vi "Configure Hardware.vi"(8 "error in (no error)":errorcluster, 11 "Cluster":T1={"Camera.lvclass"=refnum, "InClusTiming 2"={"Pixelclock"=24, "Exposure"=46.39115, "ExposureTimeBase"=2, "Framerate"=14.99615, "TriggerMode"=0}, "ROI"={"PosX"=0, "PosY"=0, "Width"=0, "Height"=0}, "File Path Control"=path "", "mirror.lvclass"=refnum} {"InClusTiming 2"."TriggerMode" items=["Auto", "Software", "External sequence start ", "External exposure control"]; "InClusTiming 2"."ExposureTimeBase" items=["nanoseconds", "microseconds", "milliseconds"]; "InClusTiming 2"."Pixelclock" min=1 max=400 step=1 scale=0.05915..400.0 scale format="%#.3g"; "InClusTiming 2"."Framerate" min=0.05915 max=2000.0 step=1.0 scale=0.05915..100.0 scale format="%#.3g"; "InClusTiming 2"."Exposure" min=0.05915 max=2000.0 step=1.0 scale=0.05915..100.0 scale format="%#.3g"}) -> (0 "error out":errorcluster, 2 "initialized array":sgl[][](array[numeric]) format="%.2f", 3 "Cluster 2":T1={"Camera.lvclass"=refnum, "InClusTiming 2"={"Pixelclock"=24, "Exposure"=46.39115, "ExposureTimeBase"=2, "Framerate"=14.99615, "TriggerMode"=0}, "ROI"={"PosX"=0, "PosY"=0, "Width"=0, "Height"=0}, "File Path Control"=path "", "mirror.lvclass"=refnum} {"InClusTiming 2"."TriggerMode" items=["Auto", "Software", "External sequence start ", "External exposure control"]; "InClusTiming 2"."ExposureTimeBase" items=["nanoseconds", "microseconds", "milliseconds"]; "InClusTiming 2"."Pixelclock" min=1 max=400 step=1 scale=0.05915..400.0 scale format="%#.3g"; "InClusTiming 2"."Framerate" min=0.05915 max=2000.0 step=1.0 scale=0.05915..100.0 scale format="%#.3g"; "InClusTiming 2"."Exposure" min=0.05915 max=2000.0 step=1.0 scale=0.05915..100.0 scale format="%#.3g"})   [LabVIEW 2020, in "Acquisition.lvlib"]
doc: "Configure the hardware."
uses:
  Acquisition.lvlib
  HardwareConfiguration.ctl
  CLASS/Image Acquisition Class/Camera.lvclass
  MIRROR/mirror.lvclass
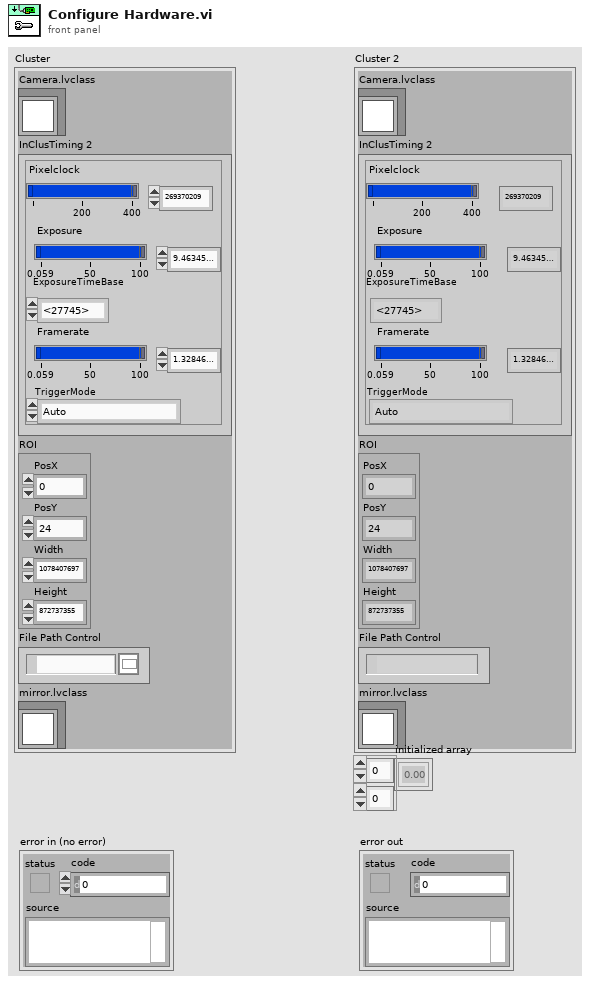
[diagram p1: front panel]
types:
  T1 = typedef "Acquisition.lvlib/HardwareConfiguration.ctl" = cluster{"Camera.lvclass":refnum<class "Camera.lvclass">, "InClusTiming 2":cluster{"Pixelclock":i32, "Exposure":dbl, "ExposureTimeBase":u16, "Framerate":dbl, "TriggerMode":u16}, "ROI":cluster{"PosX":i32, "PosY":i32, "Width":i32, "Height":i32}, "File Path Control":path, "mirror.lvclass":refnum<class "mirror.lvclass">}
  T2 = enum16{"Initialisation", "Calcul CdG a", "Calcul CdG b"}
  T3 = cluster{"Pixelclock":i32, "Exposure":dbl, "ExposureTimeBase":u16, "Framerate":dbl, "TriggerMode":u16}
  T4 = cluster{"PosX":i32, "PosY":i32, "Width":i32, "Height":i32}
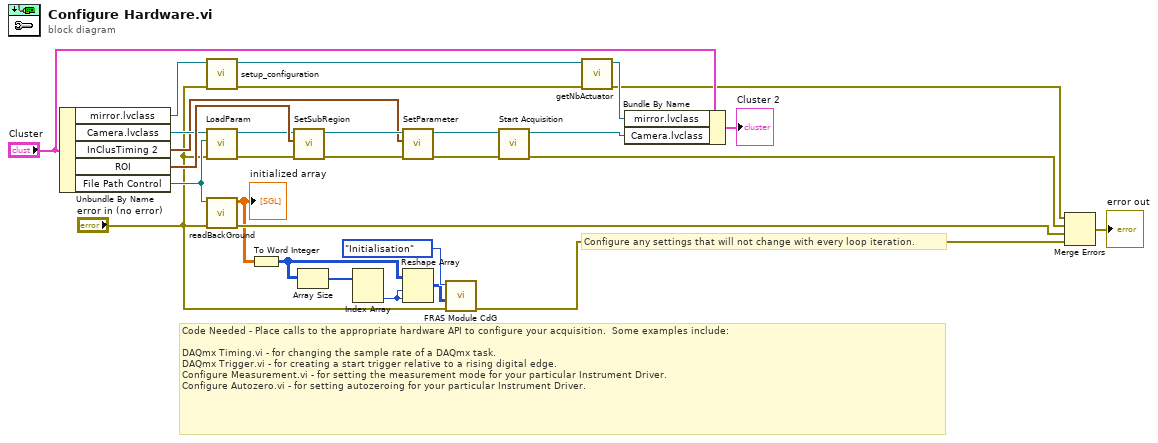
[diagram p0: block diagram]
diagram:
  # "Configure any settings that will not change with every loop iteration."
  # "Code Needed - Place calls to the appropriate hardware API to configure your acquisition.  Some examples include:\n\nDAQmx Timing.vi - for changing the sample rate of a DAQmx task.\nDAQmx Trigger.vi - for creating a start trigger relative to a rising digital edge.\nConfigure Measurement.vi - for setting the measurement mode for your particular Instrument Driver.\nConfigure Autozero.vi - for setting autozeroing for your particular Instrument Driver."
  n1 = Unbundle By Name("Cluster") -> ("mirror.lvclass"=w3:refnum<class "mirror.lvclass">, "Camera.lvclass"=w20:refnum<class "Camera.lvclass">, "InClusTiming 2"=w18:T3, "ROI"=w22:T4, "File Path Control"=w17:path)
  n2 = call-dynamic "setup_configuration.vi"("error in (no error)"="error in (no error)", "mirror in"=w3) -> ("error out"=w6:errorcluster, "mirror out"=w5:refnum<class "mirror.lvclass">)  [unwired: 8 in]
  n3 = call-dynamic "LoadParam.vi"("error in (no error)"="error in (no error)", "File Path Control"=w17, "Camera in"=w20) -> ("error out"=w21:errorcluster, "Camera out"=w19:refnum<class "Camera.lvclass">)  [unwired: 7 in]
  n4 = call "readBackGround.vi"("error in (no error)"="error in (no error)", "file (use dialog)"=w17) -> ("error out"=w16:errorcluster, "initialized array"=w11:sgl[][])  [unwired: 8 in]
  "initialized array" <- w11
  n5 = To Word Integer(number=w11) -> (16bit integer=w9:i16[][])
  n6 = call-dynamic "SetSubRegion.vi"("error in (no error)"=w21, "ROI"=w22, "Camera in"=w19) -> ("error out"=w24:errorcluster, "Camera out"=w23:refnum<class "Camera.lvclass">)  [unwired: 7 in]
  n7 = Array Size(array=w9) -> (size(s)=w8:i32[])
  n8 = Index Array(array=w8) -> (element #2=w7:i32)  [unwired: 2 in, 1 out]
  n9 = call-dynamic "SetParameter.vi"("error in (no error)"=w24, "InClusTiming"=w18, "Camera in"=w23) -> ("error out"=w29:errorcluster, "Camera out"=w28:refnum<class "Camera.lvclass">)  [unwired: 7 in]
  n10 = Reshape Array(w9, w7, w7) -> (w10:i16[][])
  n11 = call "FRAS Module CdG.vi"("error in"="error in (no error)", "Imagette seuillée"=w10, "Mode CdG"=T2."Initialisation") -> ("error out"=w12:errorcluster)  [unwired: 6 in, 1 out]
  n12 = call-dynamic "Start Acquisition.vi"("error in (no error)"=w29, "Image Acquisition in"=w28) -> ("error out"=w15:errorcluster, "Image Acquisition out"=w25:refnum<class "Camera.lvclass">)  [unwired: 8 in]
  n13 = call-dynamic "getNbActuator.vi"("error in (no error)"=w6, "mirror in"=w5) -> ("error out"=w1:errorcluster, "mirror out"=w2:refnum<class "mirror.lvclass">)  [unwired: 7 in, 1 out]
  n14 = Bundle By Name(cluster="Cluster", "mirror.lvclass"=w2, "Camera.lvclass"=w25) -> (→"Cluster 2":T1)
  n15 = Merge Errors(w1, w15, w16, w12) -> (→"error out":errorcluster)
